vi "test3_serial.vi"() -> ()   [LabVIEW 2020]
uses:
  <vilib>/Platform/TimedLoop/XDataNode/timing_clust.ctl
  <vilib>/Platform/TimedLoop/XDataNode/nitl_modes.ctl
  <vilib>/Platform/TimedLoop/XDataNode/wakeup.ctl
  37583fcc-cec8-480d-a6d0-1da09da3d0dd.vi
  <vilib>/Instr/_visa.llb/VISA Configure Serial Port (Instr).vi
  <vilib>/platform/TimedLoop/XDataNode/XDataNode.xnode
  <vilib>/Platform/TimedLoop/XDataNode/XDNodeRunTimeDep.lvlib
panel:
  in  "Stop 2":bool
  out "concatenated string":string
  out "error out":errorcluster
  in  "VISA resource name":refnum<visa-resource-name>
  out "Send":bool
  out "Tank":dbl(slide) scale=0.0..1.0
  out "Current XY":cluster{"X":dbl, "Y":dbl}
  out "XY Graph":cluster{dbl[], dbl[]}[](graph)
  out "Move Time":u32
  out "Distance":dbl
  out "Start Time":u32
  out "Start XY":cluster{"X":dbl, "Y":dbl}
  out "Target XY":cluster{"X":dbl, "Y":dbl}
  out "Stopped":bool
  in  "Stop":bool
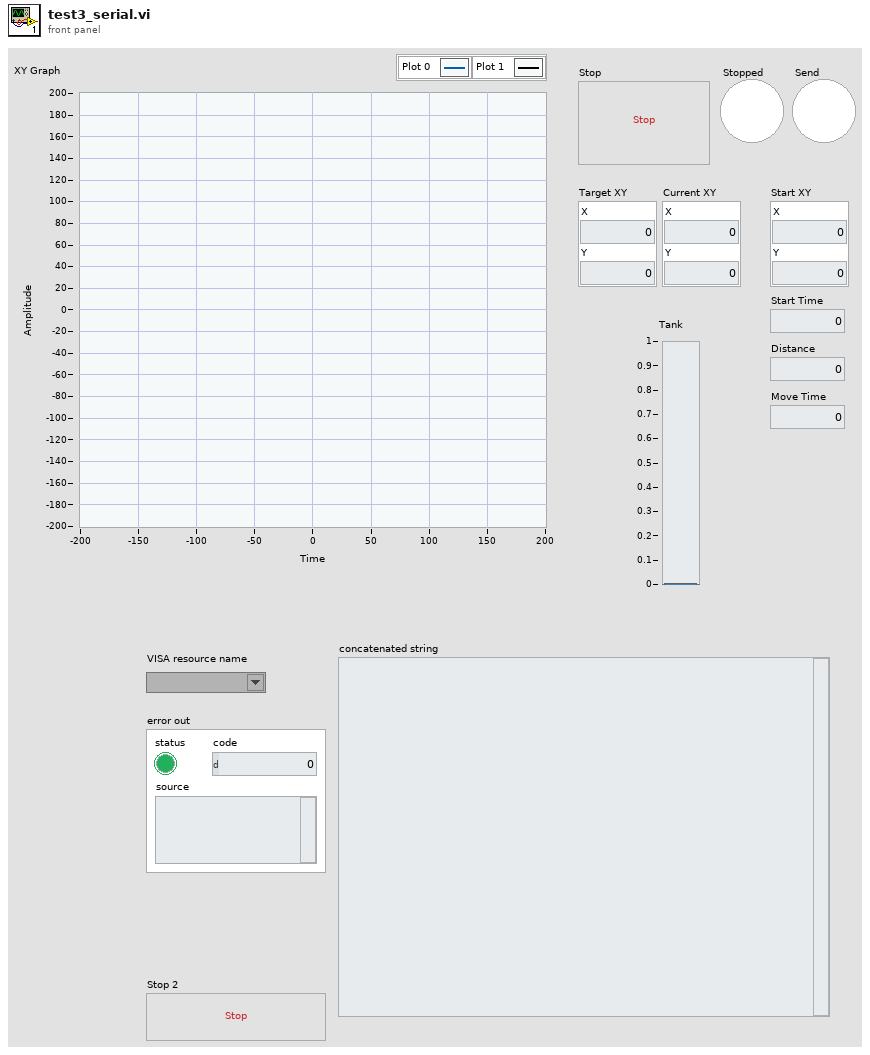
[diagram p1: front panel]
types:
  T1 = typedef "LVPoint32TypeDef.ctl" = cluster{"Horizontal":i32, "Vertical":i32}
  T2 = typedef "XDNodeRunTimeDep.lvlib/timing_clust.ctl" = cluster{"Expected End [f-1]":u64, "Actual End [f-1]":u64, "Finished Late? [f-1]":bool, "Expected End [i-1]":u64, "Actual End [i-1]":u64, "Finished Late? [i-1]":bool, "Expected Start [i]":u64, "Actual Start [i]":u64, "Expected Start [f]":u64, "Actual Start [f]":u64, "Source Name":string, "Structure Name":string, "Period":i64, "Deadline":i64, "Offset":i64, "Start":i64, "Priority":i32, "Timeout":i32, "Mode":T3, "Wakeup Reason":T4, "Error":errorcluster, "Source Type":string, "Secondary Source Type":string, "Global End Time":u64, "Global Start Time":u64, "Frame Duration":u64, "Iteration Duration":u64, "Assigned CPU":i32, "I/O Scan Engine Mode":u32}
  T3 = typedef "XDNodeRunTimeDep.lvlib/nitl_modes.ctl" = enum32{"No Change", "Process missed periods, maintain original phase", "Discard missed periods, maintain original phase", "Process missed periods, ignore original phase", "Discard missed periods, ignore original phase"}
  T4 = typedef "XDNodeRunTimeDep.lvlib/wakeup.ctl" = enum32{"Normal", "Aborted", "Asynchronous wakeup", "Timing source error", "Timed loop error", "Timeout"}
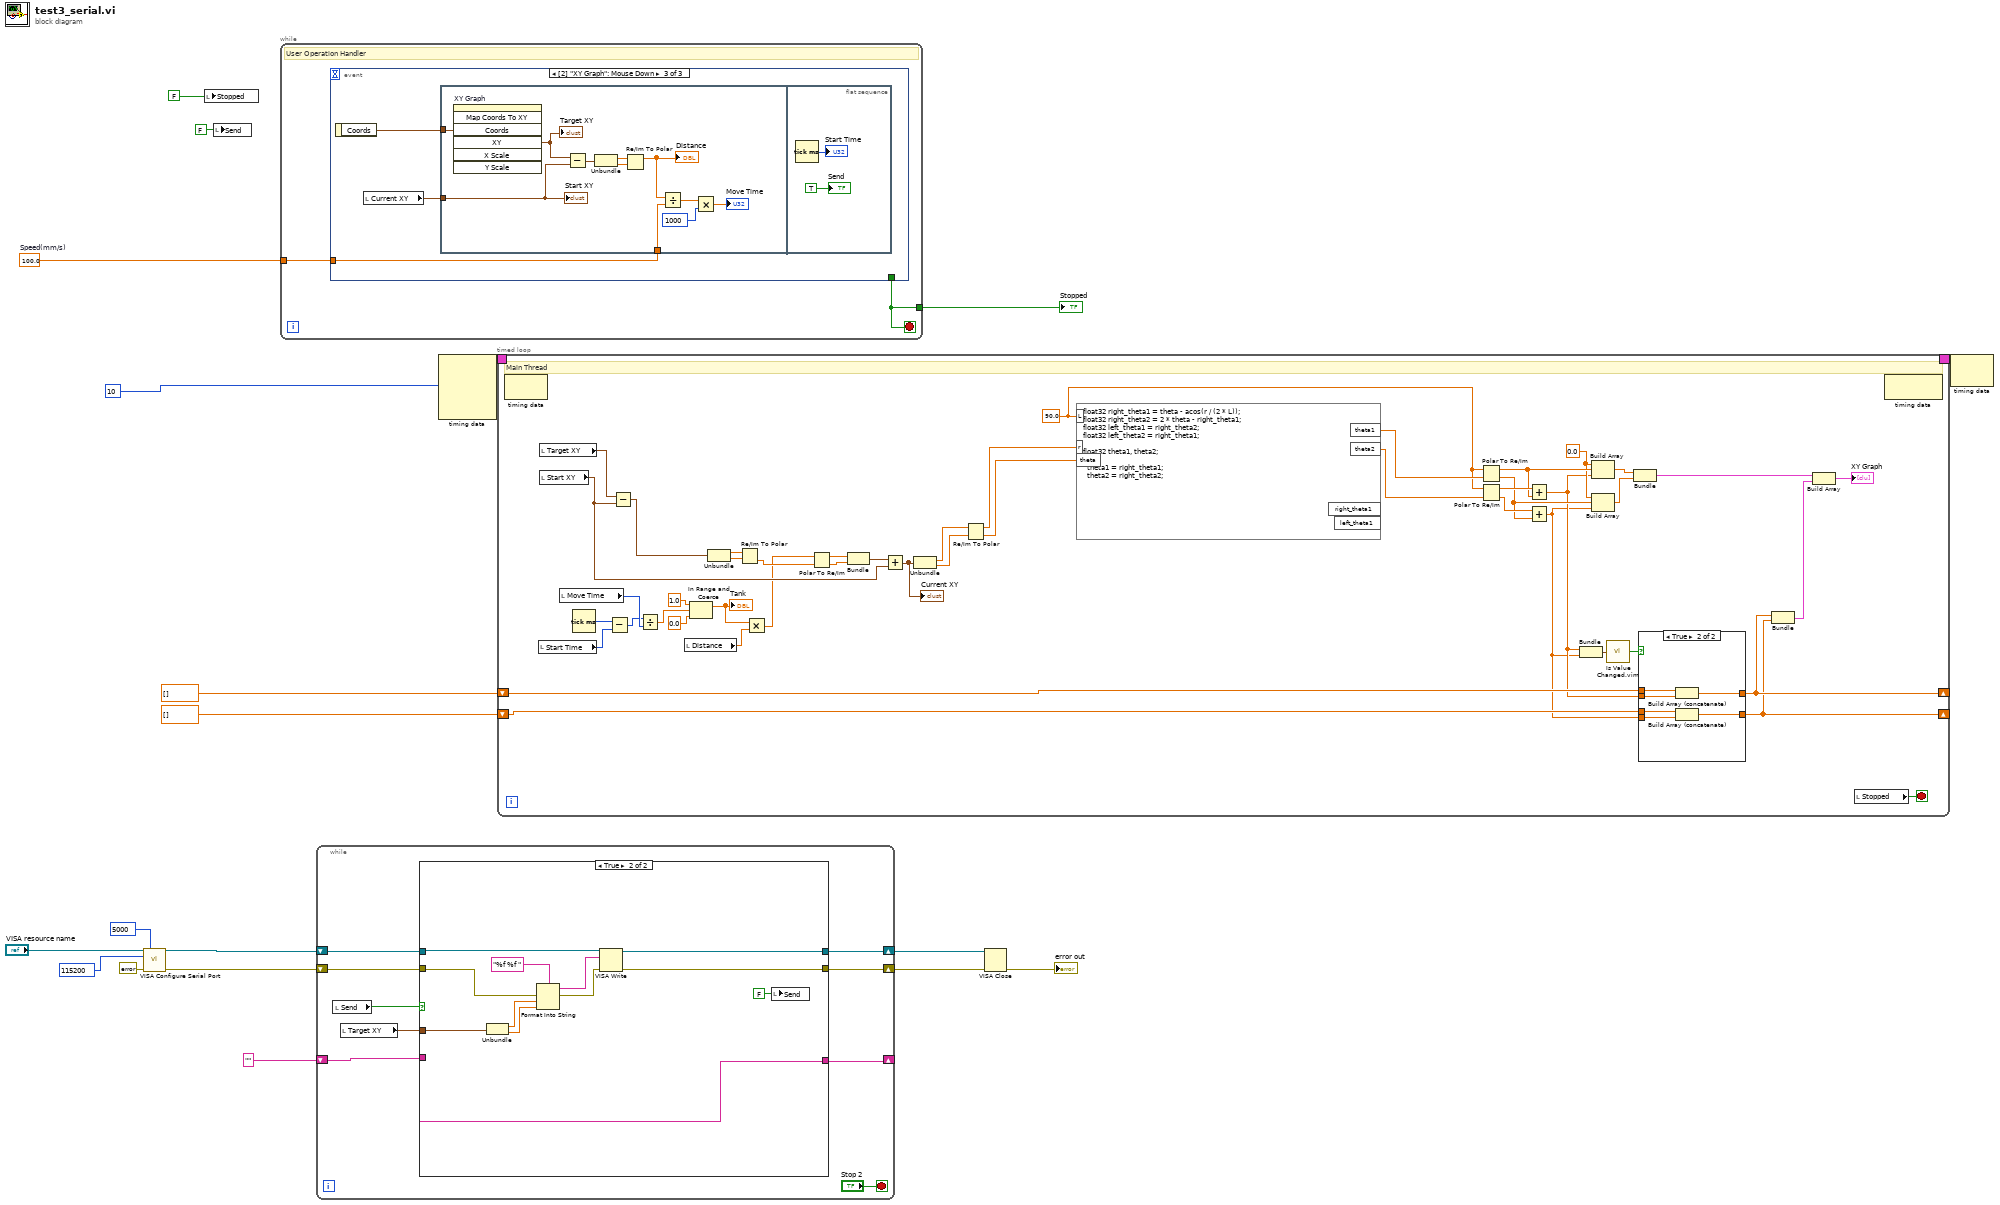
[diagram p0: block diagram]
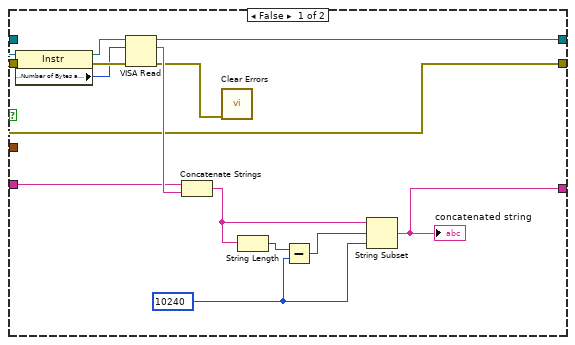
[diagram p2: hidden frame]
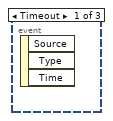
[diagram p4: hidden frame]
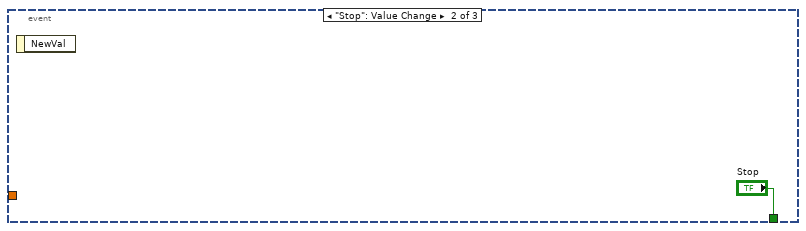
[diagram p5: hidden frame]
diagram:
  w14 = 100.0  # Speed(mm/s)
  n1 = call-poly "VISA Configure Serial Port"("VISA resource name"="VISA resource name", "timeout (10sec)"=u32 5000, "baud rate (9600)"=u32 115200, "error in (no error)"=errorcluster {"status"=FALSE, "code"=0, "source"=""}) -> ("VISA resource name out"=w7:refnum<visa-resource-name>, "error out"=w8:errorcluster)  [unwired: 10 in]
  n2 = local write "Stopped"(FALSE ("Stopped")) -> ()
  n3 = local write "Send"(FALSE ("Send")) -> ()
  n4 = while {
    tunnel: [w21] -> w17
    tunnel: w14 -> [w20]
    stop <- w21 stop-if-true
    # "User Operation Handler"
    n5 = event shown="[2] \"XY Graph\": Mouse Down" {
      selector: _ -> [_ _ _]
      dyn-events: _ -> [_ _ _]
      timeout: _ -> [_ _ _]
      tunnel: [_ "Stop" _] -> w21
      tunnel: w20 -> [_ _ w25]
      event Timeout {
        n6 = event-data() -> ()  [unwired: 1 in, 3 out]
      }
      event "Stop": Value Change {
        n7 = event-data() -> ()  [unwired: 1 in, 1 out]
      }
      event "XY Graph": Mouse Down {
        n8 = event-data() -> ("Coords"=w24:T1)  [unwired: 1 in]
        n9 = local read "Current XY"() -> (w23:cluster{"X":dbl, "Y":dbl})
        n10 = flat-sequence {
          tunnel: w25 -> [w35]
          tunnel: w24 -> [w31]
          tunnel: w23 -> [w26]
          frame #0 {
            n11 = invoke on="XY Graph" class="XYGraph (strict)" method="Map Coords To XY"("Coords"=w31) -> ("XY"=w30:cluster{"X":dbl, "Y":dbl})  [unwired: 6 in, 6 out]
            "Target XY" <- w30
            n12 = Subtract(x=w30, y=w26) -> (x-y=w29:cluster{"X":dbl, "Y":dbl})
            n13 = Unbundle(w29) -> ("X"=w28:dbl, "Y"=w27:dbl)
            n14 = Re/Im To Polar(2:w27, 3:w28) -> (1:w36:dbl)  [unwired: 1 out]
            "Distance" <- w36
            n15 = Divide(x=w36, y=w35) -> (x/y=w34:dbl)
            n16 = Multiply(x=w34, y=u32 1000 ("millisecond timer value")) -> (x*y=→"Move Time":dbl)
            "Start XY" <- w26
          }
          frame #1 {
            n17 = Tick Count (ms)() -> (millisecond timer value=→"Start Time":u32)
            "Send" <- TRUE ("Send")
          }
        }
      }
    }
  }
  "Stopped" <- w17
  n18 = while {
    shift-right: [w45] -> w6
    shift-left: w8 -> [w47]
    shift-right: [w44] -> w5
    shift-left: w7 -> [w46]
    shift-right: [w42] -> _
    shift-left: "" -> [w41]
    stop <- "Stop 2" stop-if-true
    n19 = local read "Send"() -> (w40:bool)
    n20 = local read "Target XY"() -> (w39:cluster{"X":dbl, "Y":dbl})
    n21 = case shown="True" w40 {
      tunnel: w47 -> [w53 w73]
      tunnel: w46 -> [w61 w72]
      tunnel: [w53 w71] -> w45
      tunnel: [w57 w70] -> w44
      tunnel: [w52 w69] -> w42
      tunnel: w41 -> [w55 w69]
      tunnel: w39 -> [_ w62]
      frame False {
        w49 = 10240 ("length (rest)")
        n22 = property class="Instr"(reference=w61, error in=w53) -> (reference out=w59:refnum<visa-resource-name>, error out=w60:errorcluster, "Serial Settings:Number of Bytes at Serial Port"=w58:u32)
        n23 = VISA Read(VISA resource name=w59, byte count=w58, error in (no error)=w60) -> (VISA resource name out=w57:refnum<visa-resource-name>, read buffer=w56:string, error out=w54:errorcluster)  [unwired: 1 out]
        n24 = Concatenate Strings(w55, w56) -> (w51:string)
        n25 = call <vilib>:"Clear Errors.vi"("error in (no error)"=w54) -> ()  [unwired: 5 in, 2 out]
        n26 = String Length(string=w51) -> (length=w50:i32)
        n27 = Subtract(x=w50, y=w49) -> (x-y=w48:i32)
        n28 = String Subset(string=w51, offset (0)=w48, length (rest)=w49) -> (substring=w52:string)
        "concatenated string" <- w52
      }
      frame True {
        n29 = Unbundle(w62) -> ("X"=w67:dbl, "Y"=w66:dbl)
        n30 = Format Into String(format string="%f %f ", error in=w73, w67, w66) -> (resulting string=w64:string, error out=w65:errorcluster)  [unwired: 1 in]
        n31 = VISA Write(VISA resource name=w72, write buffer=w64, error in (no error)=w65) -> (VISA resource name out=w70:refnum<visa-resource-name>, error out=w71:errorcluster)  [unwired: 1 out]
        n32 = local write "Send"(FALSE ("Send")) -> ()
      }
    }
  }
  n33 = node-c288(i64 10 ("Period")) -> (w19:T2)  [unwired: 3 in]
  n34 = timed-loop {
    timing: w19 -> [_]
    timing-out: [_] -> w18
    shift-right: [w82] -> _
    shift-left: dbl[] [] -> [w89]
    shift-right: [w81] -> _
    shift-left: dbl[] [] -> [w88]
    stop <- w119 stop-if-true
    w94 = 0.0 ("element")
    w91 = 90.0 ("input variable")
    # "Main Thread"
    n35 = node-c288() -> ()  [unwired: 1 in, 1 out]
    n36 = local read "Start Time"() -> (w117:u32)
    n37 = local read "Target XY"() -> (w116:cluster{"X":dbl, "Y":dbl})
    n38 = local read "Start XY"() -> (w107:cluster{"X":dbl, "Y":dbl})
    n39 = local read "Move Time"() -> (w103:u32)
    n40 = Tick Count (ms)() -> (millisecond timer value=w118:u32)
    n41 = Subtract(x=w118, y=w117) -> (x-y=w78:u32)
    n42 = Subtract(x=w116, y=w107) -> (x-y=w114:cluster{"X":dbl, "Y":dbl})
    n43 = Divide(x=w78, y=w103) -> (x/y=w77:dbl)
    n44 = local read "Distance"() -> (w115:dbl)
    n45 = In Range and Coerce(upper limit=1.0 ("lower limit"), x=w77, lower limit=0.0) -> (coerced(x)=w74:dbl)  [unwired: 1 out]
    "Tank" <- w74
    n46 = Unbundle(w114) -> ("X"=w113:dbl, "Y"=w112:dbl)
    n47 = Re/Im To Polar(2:w112, 3:w113) -> (0:w111:dbl)  [unwired: 1 out]
    n48 = Multiply(x=w74, y=w115) -> (x*y=w102:dbl)
    n49 = Polar To Re/Im(2:w111, 3:w102) -> (0:w109:dbl, 1:w110:dbl)
    n50 = Bundle(w110, w109) -> (w108:cluster{dbl, dbl})  [unwired: 1 in]
    n51 = Add(x=w108, y=w107) -> (x+y=w90:cluster{dbl, dbl})
    "Current XY" <- w90
    n52 = Unbundle(w90) -> (w106:dbl, w105:dbl)
    n53 = Re/Im To Polar(2:w105, 3:w106) -> (0:w104:dbl, 1:w101:dbl)
    n54 = formula code="float32 right_theta1 = theta - acos(r / (2 * L));\nfloat32 right_theta2 = 2 * theta - right_theta1;\nfloat32 left_theta1 = right_theta2;\nfloat32 left_theta2 = right_theta1;\n\nfloat32 theta1, theta2;\n\n  theta1 = right_theta1;\n  theta2 = right_theta2;"("r"=w101, "theta"=w104, "L"=w91) -> ("theta1"=w93:sgl, "theta2"=w92:sgl)  [unwired: 2 out]
    n55 = Polar To Re/Im(2:w93, 3:w91) -> (0:w97:dbl, 1:w98:dbl)
    n56 = Polar To Re/Im(2:w92, 3:w91) -> (0:w99:dbl, 1:w100:dbl)
    n57 = Add(x=w100, y=w98) -> (x+y=w87:dbl)
    n58 = Add(x=w99, y=w97) -> (x+y=w86:dbl)
    n59 = Bundle(w87, w86) -> (w85:cluster{dbl, dbl})  [unwired: 1 in]
    n60 = Build Array(w94, w98, w87) -> (w96:dbl[])
    n61 = Build Array(w94, w97, w86) -> (w95:dbl[])
    n62 = call "Is Value Changed.vim"("value"=w85) -> ("changed or first call?"=w84:bool)
    n63 = Bundle(w96, w95) -> (w83:cluster{dbl[], dbl[]})  [unwired: 1 in]
    n64 = case shown="True" w84 {
      tunnel: w87 -> [_ w127]
      tunnel: w86 -> [_ w126]
      tunnel: [w121 w125] -> w82
      tunnel: [w120 w124] -> w81
      tunnel: w89 -> [w121 w123]
      tunnel: w88 -> [w120 w122]
      frame False {
      }
      frame True {
        n65 = Build Array (concatenate)(w123, w127) -> (w125:dbl[])
        n66 = Build Array (concatenate)(w122, w126) -> (w124:dbl[])
      }
    }
    n67 = Bundle(w82, w81) -> (w80:cluster{dbl[], dbl[]})  [unwired: 1 in]
    n68 = Build Array(w83, w80) -> (→"XY Graph":cluster{dbl[], dbl[]}[])
    n69 = local read "Stopped"() -> (w119:bool)
    n70 = node-c288() -> ()  [unwired: 1 in, 1 out]
  }
  n71 = VISA Close(VISA resource name=w5, error in (no error)=w6) -> (error out=→"error out":errorcluster)
  n72 = node-c288(w18) -> ()  [unwired: 1 out]
